vi "ABB motor test Main.vi"() -> ()   [LabVIEW 2017]
uses:
  ABB global.vi
panel:
  in  "Configure":bool caption="Bearing run"
  in  "Efficiency":bool caption="Bearing run"
  in  "High Voltage test":bool caption="Bearing run"
  in  "Bearing inspection":bool caption="Bearing run"
  in  "View Report":bool caption="Bearing run"
  in  "Noise Test":bool caption="Bearing run"
  in  "Bearing run":bool
  in  "Enter Motor data":bool
  in  "Heat run":bool
  in  "Locked Rotor test":bool
  in  "No load Test":bool
  in  "Quit":bool
  # "MOTOR TEST"
  # "v3.96"
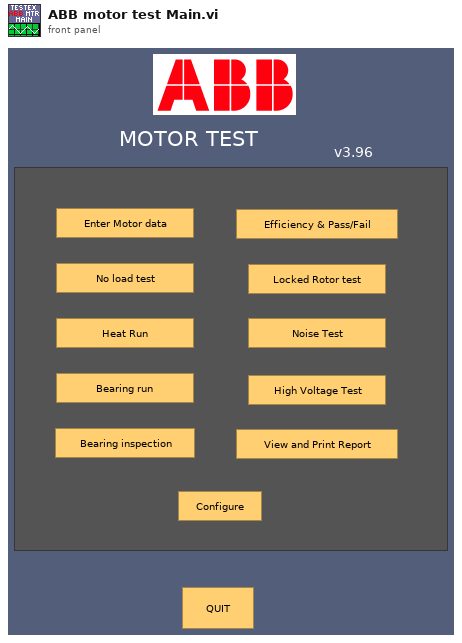
[diagram p1: front panel]
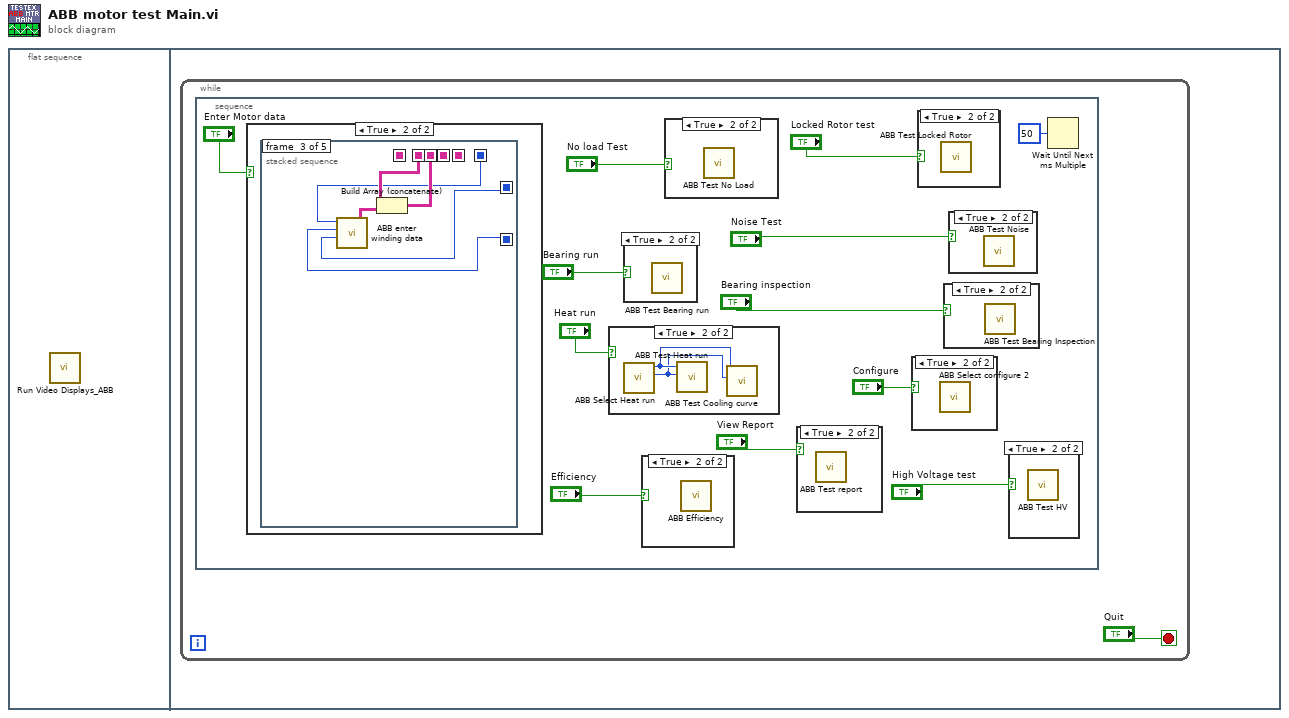
[diagram p0: block diagram]
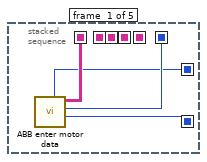
[diagram p12: hidden frame]
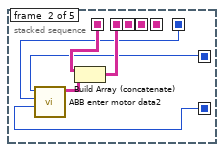
[diagram p13: hidden frame]
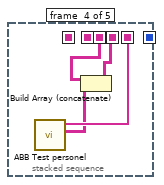
[diagram p14: hidden frame]
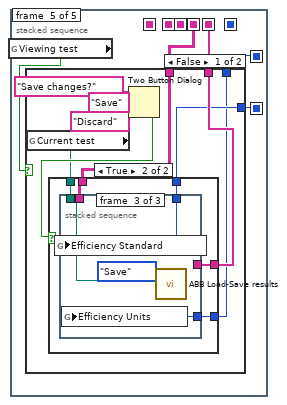
[diagram p15: hidden frame]
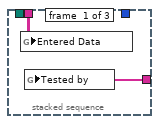
[diagram p17: hidden frame]
diagram:
  n1 = flat-sequence {
    frame #0 {
      n2 = call "Run Video Displays_ABB.vi"() -> ()  [unwired: 12 in]
    }
    frame #1 {
      n3 = while {
        stop <- "Quit" stop-if-true
        n4 = stacked-sequence {
          frame #0 {
            n5 = case shown="True" "Enter Motor data" {
              frame False {
              }
              frame True {
                n6 = stacked-sequence {
                  seq-local: [w19 _ _ _ _] -> [_ w23 _ _ _]
                  seq-local: [_ w24 _ _ _] -> [_ _ w30 _ _]
                  seq-local: [_ _ _ w35 _] -> [_ _ _ _ w39]
                  seq-local: [_ _ w29 _ _] -> [_ _ _ w33 _]
                  seq-local: [_ _ _ w32 _] -> [_ _ _ _ w38]
                  seq-local: [w18 _ _ _ _] -> [_ w22 w28 _ _]
                  seq-local: [w17 _ _ _ _] -> [_ w21 w27 _ w37]
                  seq-local: [w16 _ _ _ _] -> [_ w20 w26 _ w36]
                  frame #0 {
                    n7 = call "ABB enter motor data.vi"() -> ("Efficiency Standard out"=w17:u16, "Motor Type out"=w18:u16, "Entered data"=w19:string[][], "Efficiency Units out"=w16:u16)  [unwired: 8 in]
                  }
                  frame #1 {
                    n8 = call "ABB enter motor data2.vi"("Efficiency Standard"=w21, "Motor Type"=w22, "Efficiency Units"=w20) -> ("entered data"=w25:string[][])  [unwired: 8 in]
                    n9 = Build Array (concatenate)(w23, w25) -> (w24:string[][])
                  }
                  frame #2 {
                    n10 = call "ABB enter winding data.vi"("Efficiency Units"=w26, "Efficiency Standard"=w27, "Motor Type"=w28) -> ("entered data"=w31:string[][])  [unwired: 8 in]
                    n11 = Build Array (concatenate)(w30, w31) -> (w29:string[][])
                  }
                  frame #3 {
                    n12 = call "ABB Test personel.vi"() -> ("Attendance data"=w34:string[][], "Personel out"=w35:string[])  [unwired: 10 in]
                    n13 = Build Array (concatenate)(w33, w34) -> (w32:string[][])
                  }
                  frame #4 {
                    n14 = global read "ABB global.vi" "Viewing test"() -> (w40:bool)
                    n15 = case shown="False" w40 {
                      tunnel: w38 -> [w47 _]
                      tunnel: w39 -> [w45 _]
                      tunnel: w37 -> [w42 _]
                      tunnel: w36 -> [w41 _]
                      frame False {
                        n16 = global read "ABB global.vi" "Current test"() -> (w46:path)
                        n17 = Two Button Dialog(message="Save changes?", 1:"Discard" ("F button name (\"Cancel\")"), 2:"Save" ("T button name (\"OK\")")) -> (T button?=w48:bool)
                        n18 = case shown="True" w48 {
                          tunnel: w47 -> [_ w54]
                          tunnel: w46 -> [_ w53]
                          tunnel: w45 -> [_ w52]
                          tunnel: w42 -> [_ w51]
                          tunnel: w41 -> [_ w50]
                          frame False {
                          }
                          frame True {
                            n19 = stacked-sequence {
                              tunnel: w54 -> [w56 _ _]
                              tunnel: w53 -> [_ _ w59]
                              tunnel: w52 -> [w55 _ _]
                              tunnel: w51 -> [_ _ w58]
                              tunnel: w50 -> [_ _ w57]
                              frame #0 {
                                n20 = global write "ABB global.vi" "Entered Data"(w56) -> ()
                                n21 = global write "ABB global.vi" "Tested by"(w55) -> ()
                              }
                              frame #1 {
                              }
                              frame #2 {
                                n22 = global write "ABB global.vi" "Efficiency Standard"(w58) -> ()
                                n23 = global write "ABB global.vi" "Efficiency Units"(w57) -> ()
                                n24 = call "ABB Load-Save results.vi"("Path"=w59, "Mode"=enum16{"LOAD", "Save"}."Save") -> ()  [unwired: 10 in]
                              }
                            }
                          }
                        }
                      }
                      frame True {
                      }
                    }
                  }
                }
              }
            }
            n25 = case shown="True" "Heat run" {
              frame False {
              }
              frame True {
                n26 = call "ABB Select Heat run.vi"() -> ("Measure out"=w14:enum16{"Full Load", "Partial Load", "No Load"}, "Heat run Type out"=w15:enum16{"Full Load", "Partial- & No-Load"})  [unwired: 10 in]
                n27 = call "ABB Test Heat run.vi"("Measure"=w14, "Heat run Type"=w15) -> ()  [unwired: 10 in]
                n28 = call "ABB Test Cooling curve.vi"("Measure"=w14, "Heat run Type"=w15) -> ()  [unwired: 10 in]
              }
            }
            n29 = case shown="True" "Bearing run" {
              frame False {
              }
              frame True {
                n30 = call "ABB Test Bearing run.vi"() -> ()  [unwired: 12 in]
              }
            }
            n31 = case shown="True" "Efficiency" {
              frame False {
              }
              frame True {
                n32 = call "ABB Efficiency.vi"() -> ()  [unwired: 12 in]
              }
            }
            n33 = case shown="True" "No load Test" {
              frame False {
              }
              frame True {
                n34 = call "ABB Test No Load.vi"() -> ()  [unwired: 12 in]
              }
            }
            n35 = case shown="True" "View Report" {
              frame False {
              }
              frame True {
                n36 = call "ABB Test report .vi"() -> ()  [unwired: 5 in, 1 out]
              }
            }
            n37 = case shown="True" "Configure" {
              frame False {
              }
              frame True {
                n38 = call "ABB Select configure 2.vi"() -> ()  [unwired: 12 in]
              }
            }
            n39 = case shown="True" "Locked Rotor test" {
              frame False {
              }
              frame True {
                n40 = call "ABB Test Locked Rotor.vi"() -> ()  [unwired: 1 in]
              }
            }
            n41 = case shown="True" "Bearing inspection" {
              frame False {
              }
              frame True {
                n42 = call "ABB Test Bearing Inspection.vi"() -> ()  [unwired: 1 in]
              }
            }
            n43 = case shown="True" "Noise Test" {
              frame False {
              }
              frame True {
                n44 = call "ABB Test Noise.vi"() -> ()  [unwired: 1 in]
              }
            }
            n45 = case shown="True" "High Voltage test" {
              frame False {
              }
              frame True {
                n46 = call "ABB Test HV.vi"() -> ()  [unwired: 1 in]
              }
            }
            n47 = Wait Until Next ms Multiple(millisecond multiple=u32 50) -> ()  [unwired: 1 out]
          }
        }
      }
    }
  }
